vi "Switch.vi"(4 "Numeric":i32, 7 "Operation 2":T1(ring), 8 "UnGuarded/ Guarded":enum32{"UnGuarded", "Guarded"}(radio), 9 "Radio Buttons":enum32{"Van der Paw", "Hall Effect"}(radio), 10 "Operation 3":T1(ring), 11 "VISA Refnum in":refnum<visa-resource-name>="GPIB::6") -> (3 "Close Channel List 2":string)   [LabVIEW 2018]
uses:
  <instrlib>/Keithley 3706/Keithley 3700 Series.lvlib
panel:
  in  "Operation 5":T1(ring)
  in  "Operation 4":T1(ring)
  in  "VanderPaw/Hall effect":enum32{"Radio Selection 1", "Radio Selection 2"}(radio)
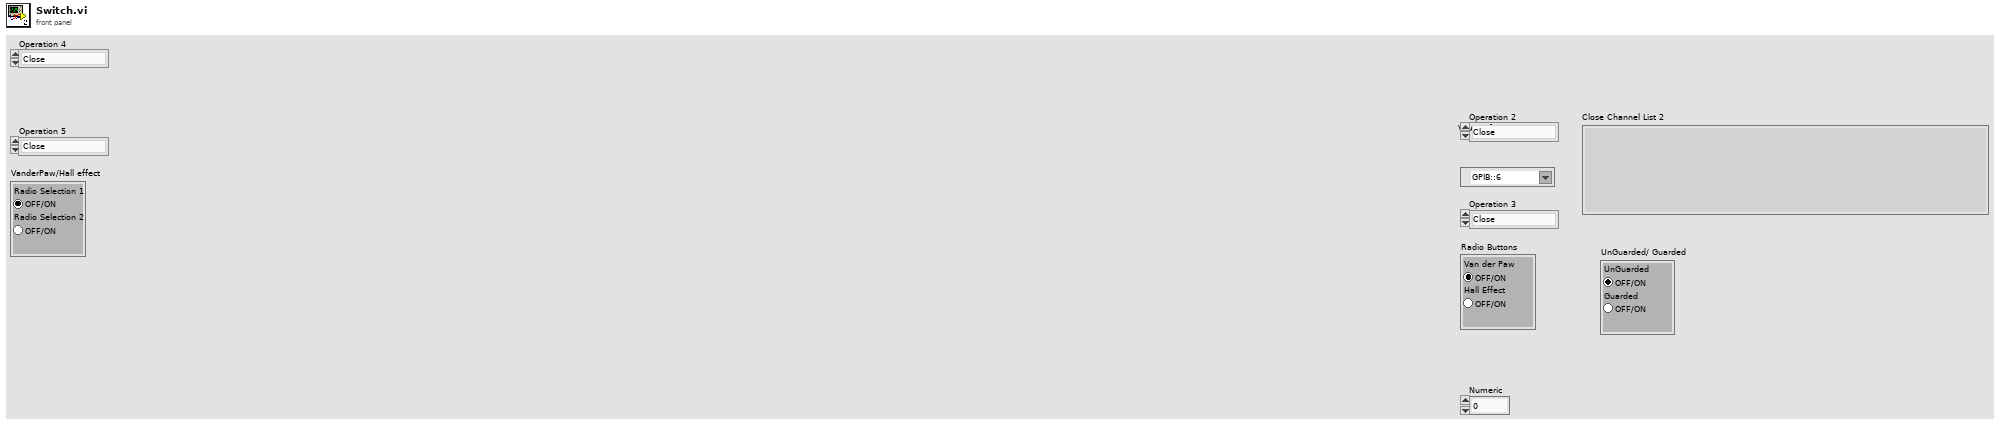
[diagram p1: front panel]
types:
  T1 = enum16{"Close", "Close Exclusive", "Close Slot Exclusive", "Open", "Open All"}
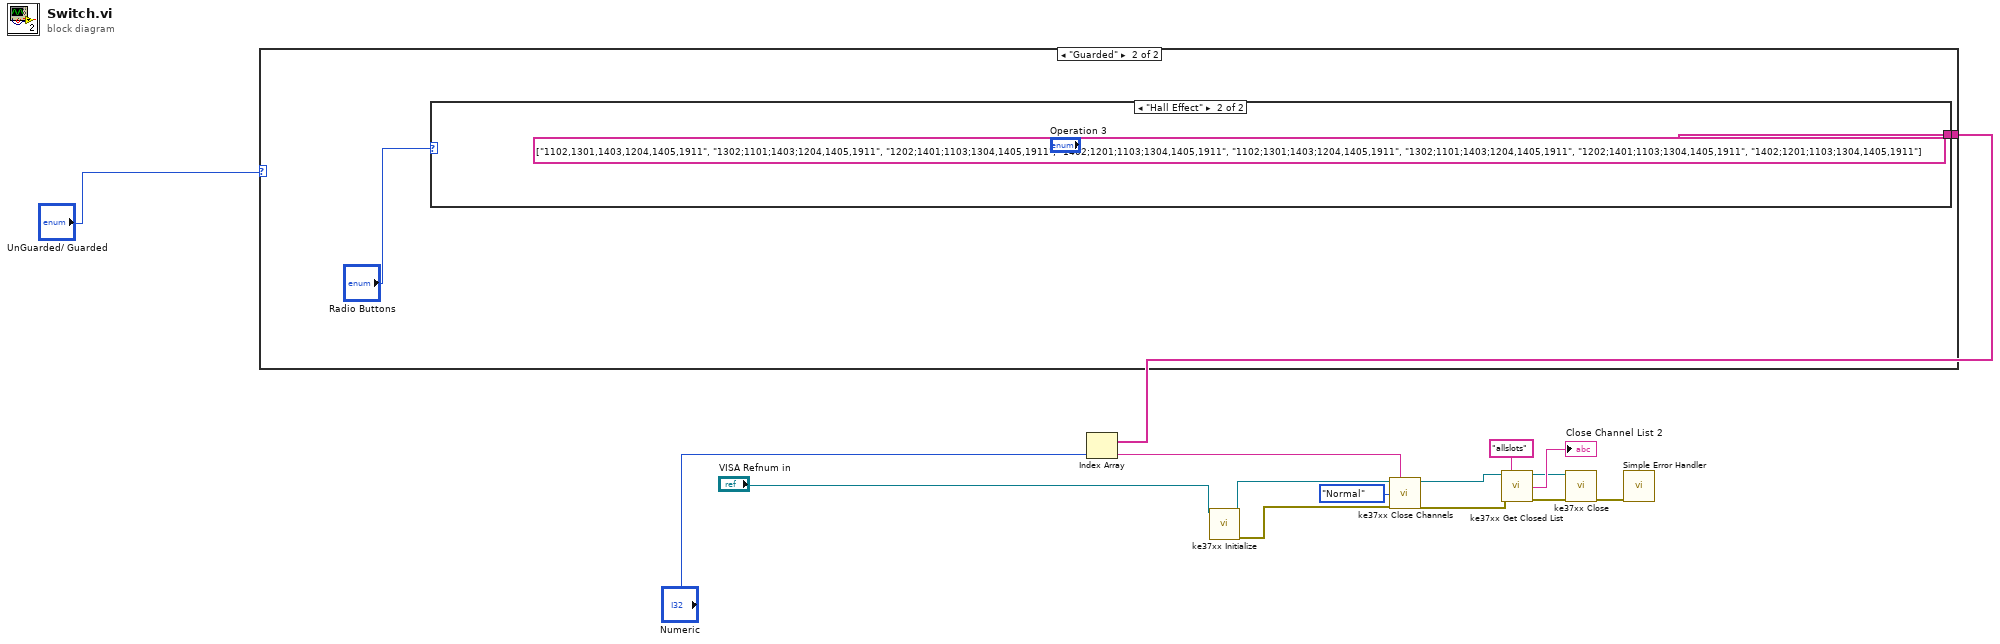
[diagram p0: block diagram]
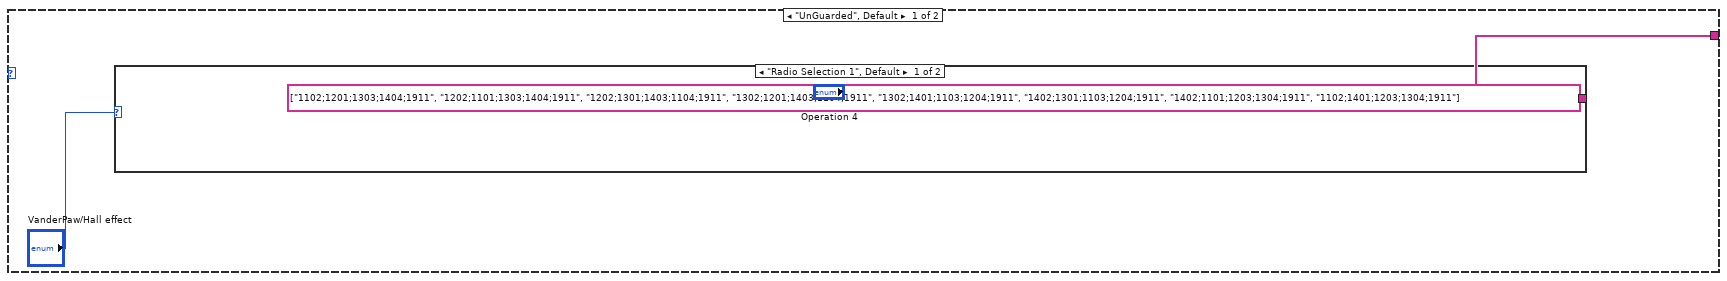
[diagram p2: hidden frame]
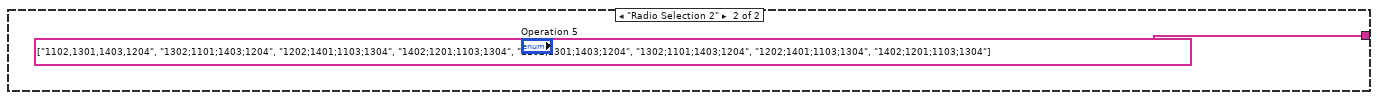
[diagram p3: hidden frame]
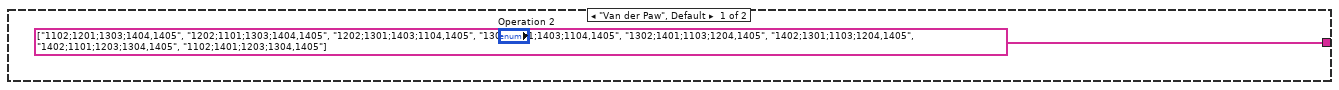
[diagram p4: hidden frame]
diagram:
  n1 = case shown="\"Guarded\"" "UnGuarded/ Guarded" {
    tunnel: [w16 w20] -> w15
    frame "UnGuarded", Default {
      n2 = case shown="\"Radio Selection 1\", Default" "VanderPaw/Hall effect" {
        tunnel: [string[] ["1102;1201;1303;1404;1911", "1202;1101;1303;1404;1911", "1202;1301;1403;1104;1911", "1302;1201;1403;1104;1911", "1302;1401;1103;1204;1911", "1402;1301;1103;1204;1911", "1402;1101;1203;1304;1911", "1102;1401;1203;1304;1911"] string[] ["1102,1301,1403,1204", "1302;1101;1403;1204", "1202;1401;1103;1304", "1402;1201;1103;1304", "1102;1301;1403;1204", "1302;1101;1403;1204", "1202;1401;1103;1304", "1402;1201;1103;1304"]] -> w16
        frame "Radio Selection 1", Default {
        }
        frame "Radio Selection 2" {
        }
      }
    }
    frame "Guarded" {
      n3 = case shown="\"Hall Effect\"" "Radio Buttons" {
        tunnel: [string[] ["1102;1201;1303;1404,1405", "1202;1101;1303;1404,1405", "1202;1301;1403;1104,1405", "1302;1201;1403;1104,1405", "1302;1401;1103;1204,1405", "1402;1301;1103;1204,1405", "1402;1101;1203;1304,1405", "1102;1401;1203;1304,1405"] string[] ["1102,1301,1403,1204,1405,1911", "1302;1101;1403;1204,1405,1911", "1202;1401;1103;1304,1405,1911", "1402;1201;1103;1304,1405,1911", "1102;1301;1403;1204,1405,1911", "1302;1101;1403;1204,1405,1911", "1202;1401;1103;1304,1405,1911", "1402;1201;1103;1304,1405,1911"]] -> w20
        frame "Van der Paw", Default {
        }
        frame "Hall Effect" {
        }
      }
    }
  }
  n4 = Index Array(array=w15, index="Numeric") -> (element=w6:string)
  n5 = call <instrlib>:"ke37xx Initialize.vi"("VISA resource name"="VISA Refnum in") -> ("VISA resource name out"=w5:refnum<visa-resource-name>, "error out"=w4:errorcluster)  [unwired: 13 in]
  n6 = call <instrlib>:"ke37xx Close Channels.vi"("VISA Resource Name"=w5, "Channel List"=w6, "Mode (0: Normal)"=enum16{"Normal", "Exclusive", "Slot Exclusive"}."Normal", "error in (no error)"=w4) -> ("VISA Resource Name Out"=w3:refnum<visa-resource-name>, "error out"=w2:errorcluster)  [unwired: 10 in]
  n7 = call <instrlib>:"ke37xx Get Closed List.vi"("VISA Resource Name"=w3, "Channel List"="allslots", "error in (no error)"=w2) -> ("VISA Resource Name Out"=w10:refnum<visa-resource-name>, "Closed List"=→"Close Channel List 2":string, "error out"=w11:errorcluster)  [unwired: 10 in]
  n8 = call <instrlib>:"ke37xx Close.vi"("VISA resource name"=w10, "error in (no error)"=w11) -> ("error out"=w9:errorcluster)  [unwired: 13 in]
  n9 = call <vilib>:"Simple Error Handler.vi"("error in (no error)"=w9) -> ()  [unwired: 1 in, 8 out]
